vi "Generate Requests.vi"(8 "trigger":bool, 11 "delays":u16[](array[numeric])) -> (3 "request":T1)   [LabVIEW 2023]
uses:
  <instrlib>/niUSRP/Reference FPGA/ZBX Control/ZBX IO Request.ctl
  <instrlib>/_niInstr/Basic Elements/v1/FPGA/Private/Count Down U16.vi
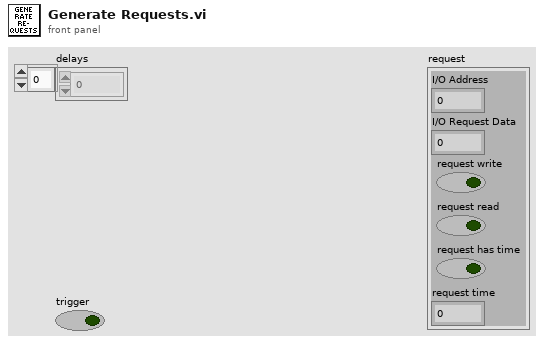
[diagram p1: front panel]
types:
  T1 = typedef "ZBX IO Request.ctl" = cluster{"I/O Address":fxp<+,20,20>, "I/O Request Data":u32, "request write":bool, "request read":bool, "request has time":bool, "request time":u64}
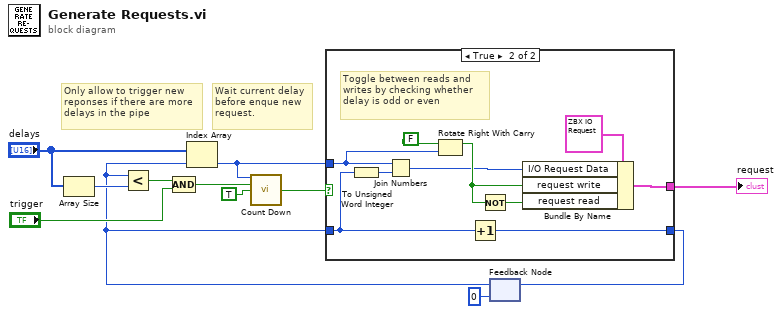
[diagram p0: block diagram]
diagram:
  # "Wait current delay\nbefore enque new\nrequest."
  # "Only allow to trigger new\nreponses if there are more\ndelays in the pipe"
  n1 = Array Size(array="delays") -> (size(s)=w4:i32)
  n2 = feedback #1(0 ("counter in")) -> (w1:i32)
  n3 = Less?(x=w1, y=w4) -> (x < y?=w7:bool)
  n4 = Compound Arithmetic op=AND(w7, "trigger") -> (w8:bool)
  n5 = Index Array(array="delays", index=w1) -> (element=w10:u16)
  n6 = call-poly <instrlib>:"Count Down.vi"("count in"=w10, "load"=w8, "decrement"=TRUE) -> ("terminal count"=w11:bool)  [unwired: 11 in, 1 out]
  n7 = case shown="True" w11 {
    tunnel: w1 -> [w13 w17]
    tunnel: [w13 w19] -> w3
    tunnel: [_ w20] -> w9
    tunnel: w10 -> [_ w15]
    frame False {
    }
    frame True {
      # "Toggle between reads and writes by checking whether delay is odd or even"
      n8 = To Unsigned Word Integer(number=w17) -> (unsigned 16bit integer=w16:u16)
      n9 = Join Numbers(hi=w15, lo=w16) -> ((hi.lo)=w18:u32)
      n10 = Rotate Right With Carry(2:w15, 3:FALSE ("carry")) -> (1:w21:bool)  [unwired: 1 out]
      n11 = Increment(x=w17) -> (x+1=w19:i32)
      n12 = Not(x=w21) -> (.not. x?=w22:bool)
      n13 = Bundle By Name(cluster=T1 {"I/O Address"=0.0, "I/O Request Data"=0, "request write"=FALSE, "request read"=FALSE, "request has time"=FALSE, "request time"=0} ("request 1"), "I/O Request Data"=w18, "request write"=w21, "request read"=w22) -> (w20:T1)
    }
  }
  "request" <- w9
  n14 = feedback-in #1(w3) -> ()
